vi "FGV_Elapsed.vi"(0 "Function":enum16{"Elapsed", "Reset"}(ring)=enum."Reset", 2 "DateTime":timestamp) -> (1 "Elapsed":dbl)   [LabVIEW 2015]
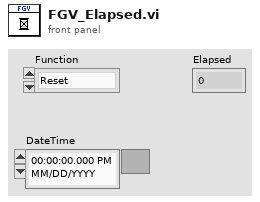
[diagram p1: front panel]
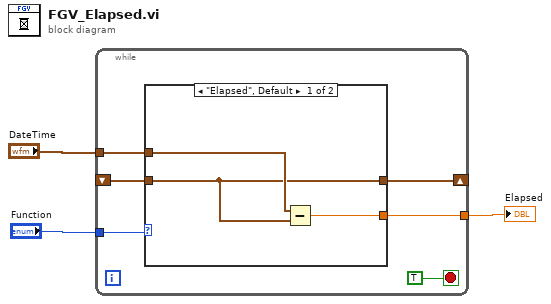
[diagram p0: block diagram]
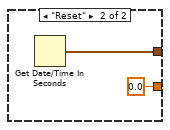
[diagram p2: hidden frame]
diagram:
  n1 = while {
    shift-right: [w7] -> _
    shift-left: _ -> [w8]
    tunnel: "Function" -> [w9]
    tunnel: [w6] -> w2
    tunnel: "DateTime" -> [w4]
    stop <- TRUE stop-if-true
    n2 = case shown="\"Elapsed\", Default" w9 {
      tunnel: w8 -> [w10 _]
      tunnel: [w10 w13] -> w7
      tunnel: [w12 0.0] -> w6
      tunnel: w4 -> [w11 _]
      frame "Elapsed", Default {
        n3 = Subtract(x=w11, y=w10) -> (x-y=w12:dbl)
      }
      frame "Reset" {
        n4 = Get Date/Time In Seconds() -> (seconds since 1Jan1904=w13:timestamp)
      }
    }
  }
  "Elapsed" <- w2
